vi "AdjustAmplifier.vi"(10 "Voltage":dbl) -> ()   [LabVIEW 2017]
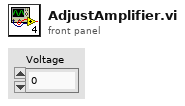
[diagram p1: front panel]
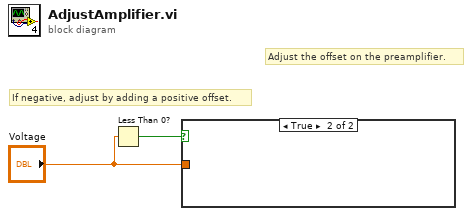
[diagram p0: block diagram]
diagram:
  # "If negative, adjust by adding a positive offset."
  # "Adjust the offset on the preamplifier."
  n1 = Less Than 0?(x="Voltage") -> (x < 0?=w2:bool)
  n2 = case shown="True" w2 {
    tunnel: "Voltage" -> [_ _]
    frame False {
    }
    frame True {
    }
  }
